vi "Point+Scan .vi"() -> ()   [LabVIEW 2014]
doc: "This is the main user interface of the Raman spectroscopy system."
uses:
  <userlib>/atmcd64d.llb/AcquisitionMode_mode typedef.ctl
  <userlib>/atmcd64d.llb/ReadMode_mode typedef.ctl
  <userlib>/atmcd64d.llb/Shutter_mode typedef.ctl
  <userlib>/atmcd64d.llb/Shutter_type typedef.ctl
  <userlib>/atmcd64d.llb/TriggerMode_mode typedef.ctl
  TypeDef/GalvoInput.ctl
  <userlib>/atmcd64d.llb/Error Code Enum typedef.ctl
  TypeDef/States.ctl
panel:
  in  "Tab Control":enum32{"Main", "Andor", "Galvo"}(tab)
  in  "Scan Range":T1={"Ver_V/H"=0.070604, "Hor_V/W"=0.086202, "Ver_r/p"=4.0, "Hor_r/p"=4.0}
  in  "Scan Resolusion":T2={"Ver_V"=0.17651, "Hor_H"=0.2155, "Ver_Pix"=471.9764, "Hor_Pix"=471.9764}
  in  "Galvo Center":bool
  out "Galvo":bool
  in  "Quit":bool
  out "Initialization finished":bool
  in  "Galvo Stop":bool
  in  "Galvo Scan":bool
  out "Andor":bool
  out "CurrentFrame":i32
  out "H":i32
  out "V":i32
  in  "Set":bool
  in  "AndorSnap":bool
  out "SaveStatus":bool
  in  "FilePath":string="C:\\Users\\light\\Desktop\\SI+Raman\\data\\TEMP"
  in  "Exit":bool
  out "ShutDown":cluster{"CoolOff":bool, "ShutDown":bool}
  in  "Mode":T8={"AcqMode"=enum."Single Scan", "ReadMode"=enum."Single-Track", "ShutterMode"=enum."Auto", "GateMode"=enum."TTL High", "TriggerMode"=enum."Internal"}
  in  "AcqSet":T9={"openingtime"=0, "closingtime/ms"=0, "ExposureTime/s"=0.1, "AccumCycTime"=0.0, "AccumCycNum"=1, "KineticNum"=1, "KineticTime"=0.0} {"KineticTime" format="%.5f"; "AccumCycNum" format="%.5f"; "AccumCycTime" format="%.5f"; "ExposureTime/s" format="%.5f"; "closingtime/ms" format="%.2f"; "openingtime" format="%.2f"}
  out "Timing":T10 {"kinetic" format="%.7f"; "accumulate" format="%.7f"; "exposure" format="%.7f"}
  out "SetOut":T11
  in  "MultiTrack":cluster{"StartRow":i32, "EndRow":i32}={"StartRow"=122, "EndRow"=133}
  out "SetStatus":bool
  out "CurrentTemp":i32
  out "DevInit":bool
  out "DevSize":cluster{"xpixels":i32, "ypixels":i32}
  out "HardWVersion":T12
  out "SoftWVersion":T13
  out "Speeds":T14
  in  "TargetTemp":i32=-60
  out "CoolerON":T15
  out "GetStatus":T16
  in  "YOffset":dbl=5.75 caption="Offset"
  in  "XOffset":dbl=3.1 caption="Offset"
  out "Sample Rate":dbl=1000.0 format="%0.2f"
  out "Waveform Graph":waveform(dbl)[](graph)=[{"t0"=timestamp(0 s since 1904-01-01), "dt"=0.001, "Y"=[]}]
  in  "ZOffset":dbl=1.6 caption="Offset"
  in  "Galvo":T17={"Sample Rate"=100000.0, "Sample Clock Source"="OnboardClock", "Max Voltage"=10.0, "Min Voltage"=-10.0, "Physical Channel(s)"="Dev1/ao0,Dev1/ao1,Dev1/ao3"}
  # "Objective: CFI Plan Fluor ELWD 60x (1.27 NA) \nThe depth of field: 1.78 um\nPixel Size: 0.0877um/px"
  # "Kinetics->SignleTrack"
  # "Galvo Control"
  # "50Hz->1s"
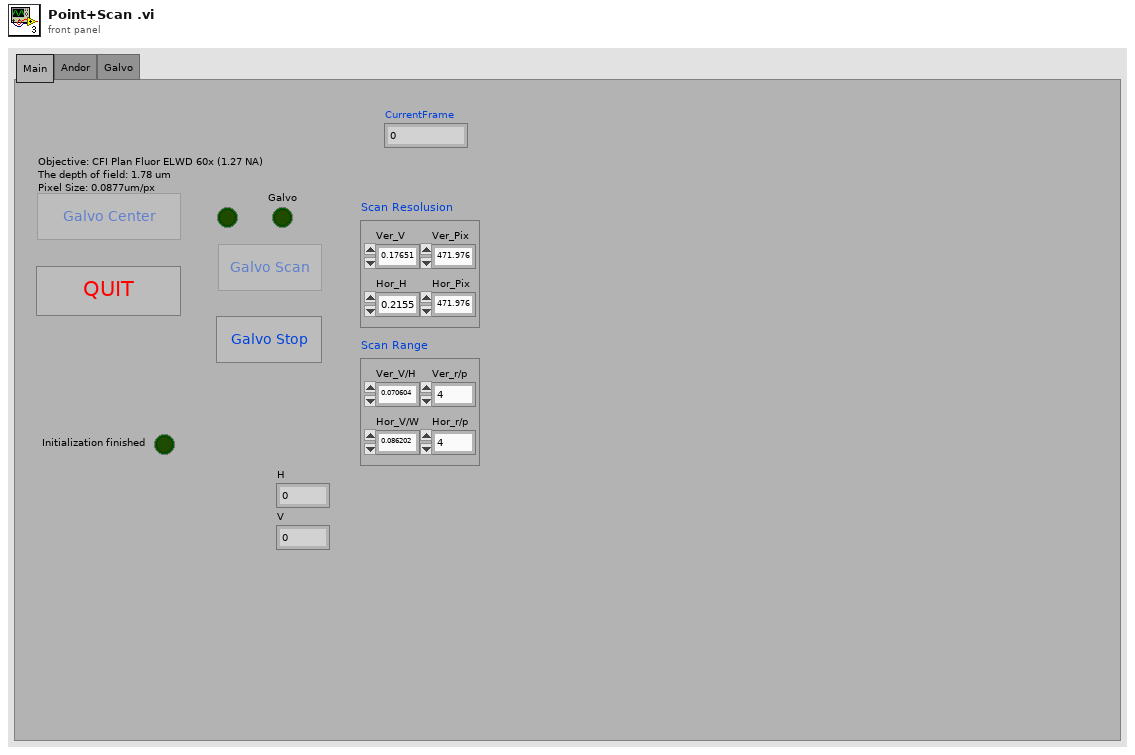
[diagram p1: front panel]
types:
  T1 = cluster{"Ver_V/H":dbl, "Hor_V/W":dbl, "Ver_r/p":dbl, "Hor_r/p":dbl}
  T2 = cluster{"Ver_V":dbl, "Hor_H":dbl, "Ver_Pix":dbl, "Hor_Pix":dbl}
  T3 = typedef "AcquisitionMode_mode typedef.ctl" = enum16{"Reserved (0)", "Single Scan", "Accumulate", "Kinetics", "Fast Kinetics", "Run Till Abort", "Reserved (6)", "Reserved (7)", "Reserved (8)", "Time Delayed Integration"}
  T4 = typedef "ReadMode_mode typedef.ctl" = enum16{"Full Vertical Binning", "Multi-Track", "Random-Track", "Single-Track", "Image"}
  T5 = typedef "Shutter_mode typedef.ctl" = enum16{"Auto", "Open", "Close", "N/A (3)", "Open FVB Series", "Open Any Series"}
  T6 = typedef "Shutter_type typedef.ctl" = enum16{"TTL Low", "TTL High"}
  T7 = typedef "TriggerMode_mode typedef.ctl" = enum16{"Internal", "External", "N/A (2)", "N/A (3)", "N/A (4)", "N/A (5)", "External Start", "External Exposure (Bulb)", "N/A (8)", "External FVB EM", "Software", "N/A (11)", "External Charge Shifting"}
  T8 = cluster{"AcqMode":T3, "ReadMode":T4, "ShutterMode":T5, "GateMode":T6, "TriggerMode":T7}
  T9 = cluster{"openingtime":i32, "closingtime/ms":i32, "ExposureTime/s":sgl, "AccumCycTime":sgl, "AccumCycNum":i32, "KineticNum":i32, "KineticTime":sgl}
  T10 = cluster{"exposure":sgl, "accumulate":sgl, "kinetic":sgl}
  T11 = cluster{"Height":i32, "Width":i32, "bottom":i32, "gap":i32}
  T12 = cluster{"PCB":u32, "Flex":u32, "dummy1":u32, "dummy2":u32, "dummy3":u32, "dummy4":u32}
  T13 = cluster{"eprom":u32, "cofFile":u32, "vxdRev":u32, "vxdVer":u32, "dllRev":u32, "dllVer":u32}
  T14 = cluster{"NVS":i32, "VS":i32, "NHS":dbl, "HS":i32}
  T15 = cluster{"SetTemp":bool, "CoolerOn":bool, "Stablized":bool}
  T16 = cluster{"GetDetector":bool, "GetHardVer":bool, "GetNVS":bool, "GetVS":bool, "GetSotfVer":bool, "GetNHS":bool, "GetHS":bool}
  T17 = typedef "GalvoInput.ctl" = cluster{"Sample Rate":dbl, "Sample Clock Source":tag, "Max Voltage":dbl, "Min Voltage":dbl, "Physical Channel(s)":tag}
  T18 = typedef "States.ctl" = enum16{"Initialize", "CMOS live", "Shut down"}
  T19 = enum8{"Enabled", "Disabled", "Disabled and Grayed Out"}
  T20 = typedef "Error Code Enum typedef.ctl" = enum32{"N/A (0)", "DRV_ERROR_CODES", "DRV_SUCCESS", "DRV_VXDNOTINSTALLED", "DRV_ERROR_SCAN", "DRV_ERROR_CHECK_SUM", "DRV_ERROR_FILELOAD", "DRV_UNKNOWN_FUNC", "DRV_ERROR_VXD_INIT", "DRV_ERROR_ADDRESS", "DRV_ERROR_PAGELOCK", "DRV_ERROR_PAGEUNLOCK", "DRV_ERROR_BOARDTEST", "DRV_ERROR_ACK", "DRV_ERROR_UP_FIFO", "DRV_ERROR_PATTERN", "N/A (16)", "DRV_ACQUISITION_ERRORS", "DRV_ACQ_BUFFER", "DRV_ACQ_DOWNFIFO_FULL", "DRV_PROC_UNKONWN_INSTRUCTION", "DRV_ILLEGAL_OP_CODE", "DRV_KINETIC_TIME_NOT_MET", "DRV_ACCUM_TIME_NOT_MET", "DRV_NO_NEW_DATA", "N/A (25)", "DRV_SPOOLERROR", "N/A (27)", "N/A (28)", "N/A (29)", "N/A (30)", "N/A (31)", "N/A (32)", "DRV_TEMPERATURE_CODES", "DRV_TEMPERATURE_OFF", "DRV_TEMPERATURE_NOT_STABILIZED", "DRV_TEMPERATURE_STABILIZED", "DRV_TEMPERATURE_NOT_REACHED", "DRV_TEMPERATURE_OUT_RANGE", "DRV_TEMPERATURE_NOT_SUPPORTED", "DRV_TEMPERATURE_DRIFT", "N/A (41)", "N/A (42)", "N/A (43)", "N/A (44)", "N/A (45)", "N/A (46)", "N/A (47)", "N/A (48)", "DRV_GENERAL_ERRORS", "DRV_INVALID_AUX", "DRV_COF_NOTLOADED", "DRV_FPGAPROG", "DRV_FLEXERROR", "DRV_GPIBERROR", "N/A (55)", "N/A (56)", "N/A (57)", "N/A (58)", "N/A (59)", "N/A (60)", "N/A (61)", "N/A (62)", "N/A (63)", "DRV_DATATYPE", "DRV_DRIVER_ERRORS", "DRV_P1INVALID", "DRV_P2INVALID", "DRV_P3INVALID", "DRV_P4INVALID", "DRV_INIERROR", "DRV_COFERROR", "DRV_ACQUIRING", "DRV_IDLE", "DRV_TEMPCYCLE", "DRV_NOT_INITIALIZED", "DRV_P5INVALID", "DRV_P6INVALID", "DRV_INVALID_MODE", "DRV_INVALID_FILTER", "DRV_I2CERRORS", "DRV_I2CDEVNOTFOUND", "DRV_I2CTIMEOUT", "DRV_P7INVALID", "N/A (84)", "N/A (85)", "N/A (86)", "N/A (87)", "N/A (88)", "N/A (89)", "DRV_IOCERROR", "DRV_VRMVERSIONERROR"}
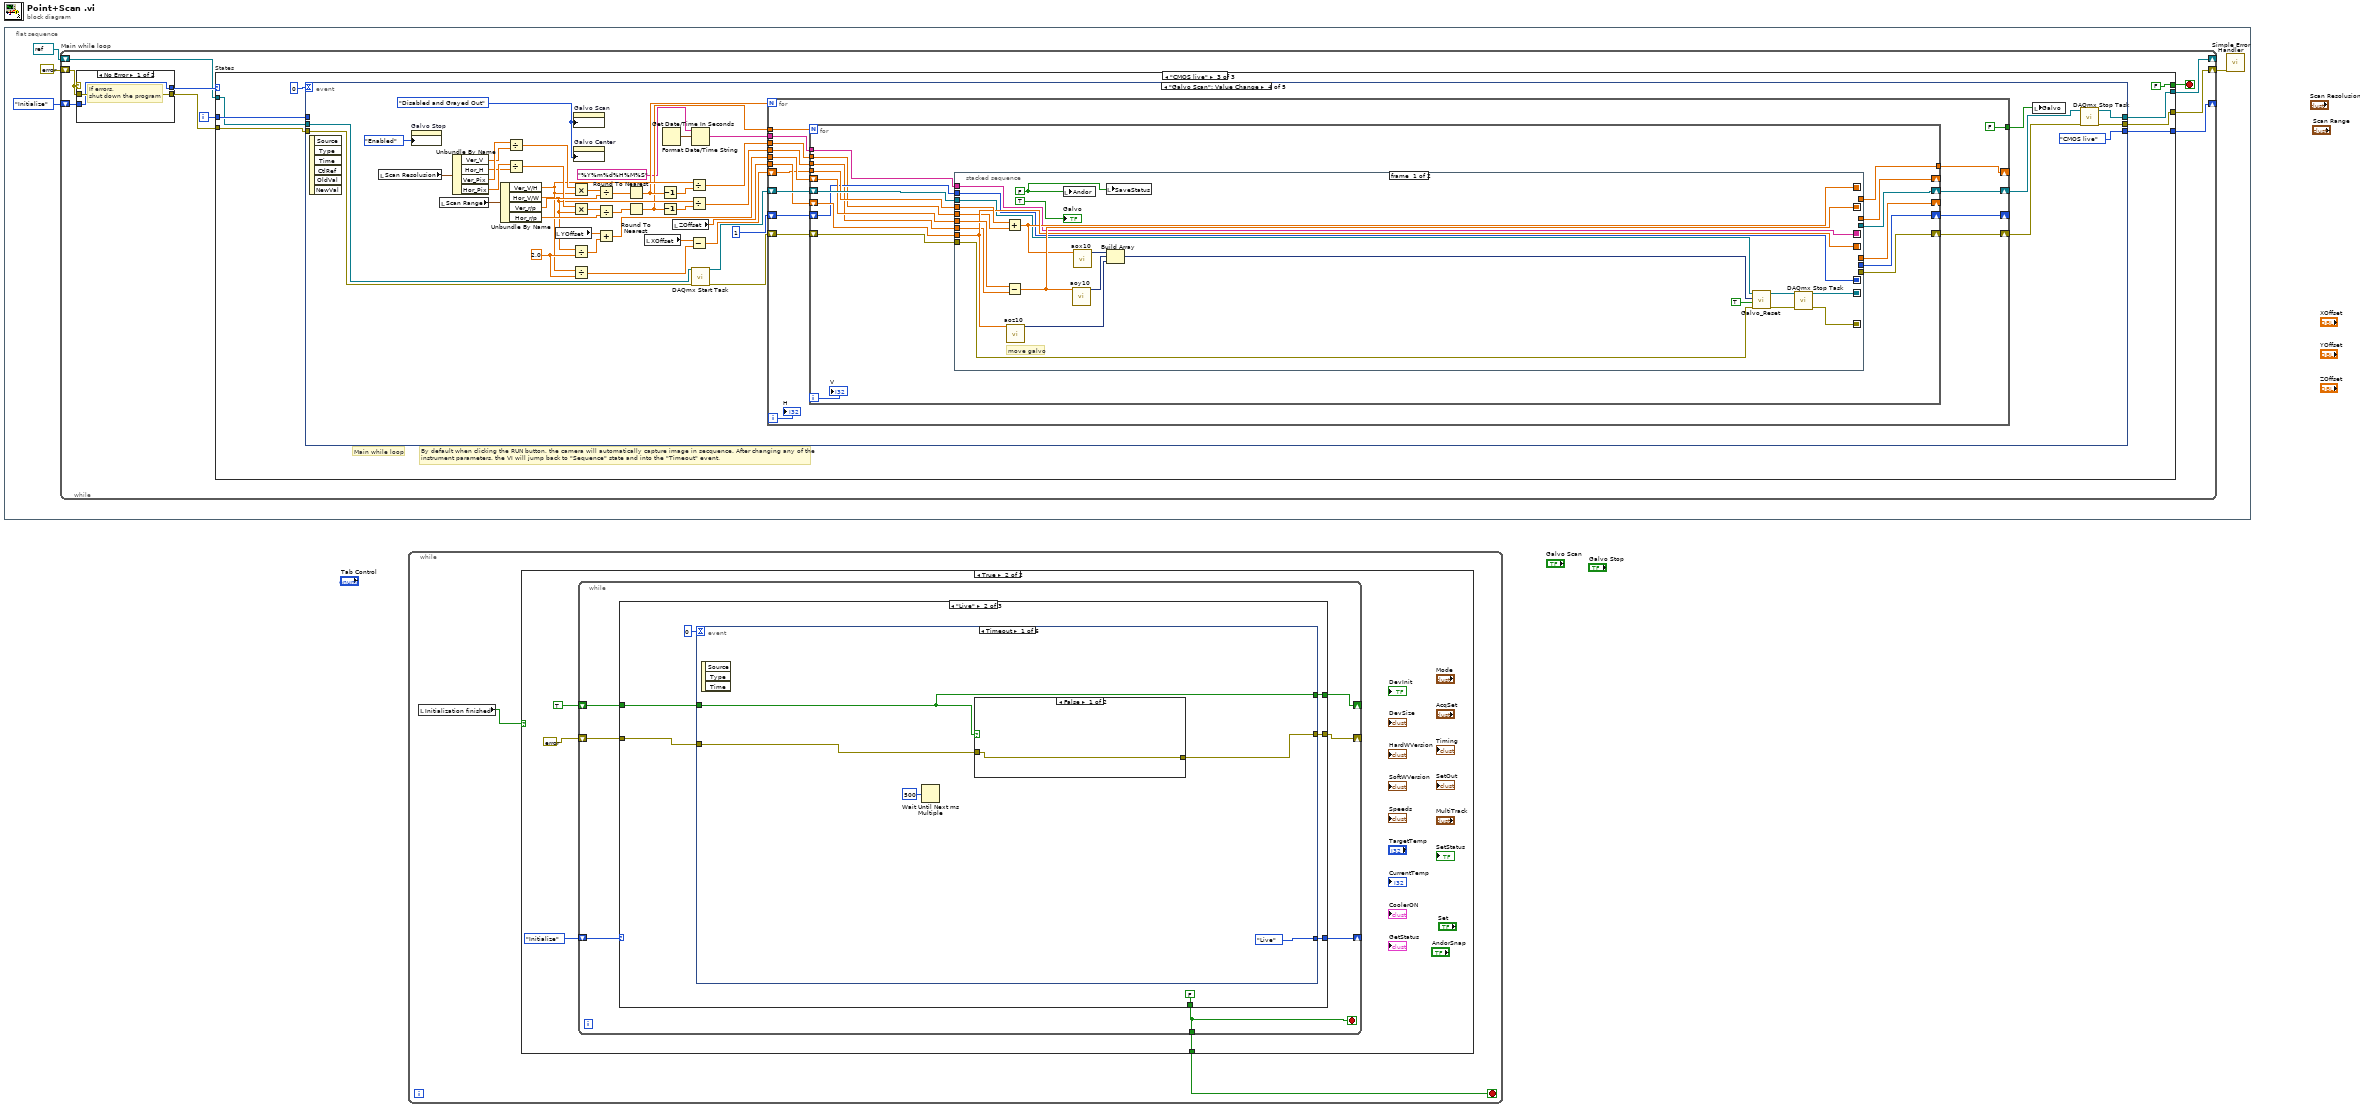
[diagram p0: block diagram]
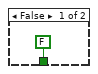
[diagram p2: hidden frame]
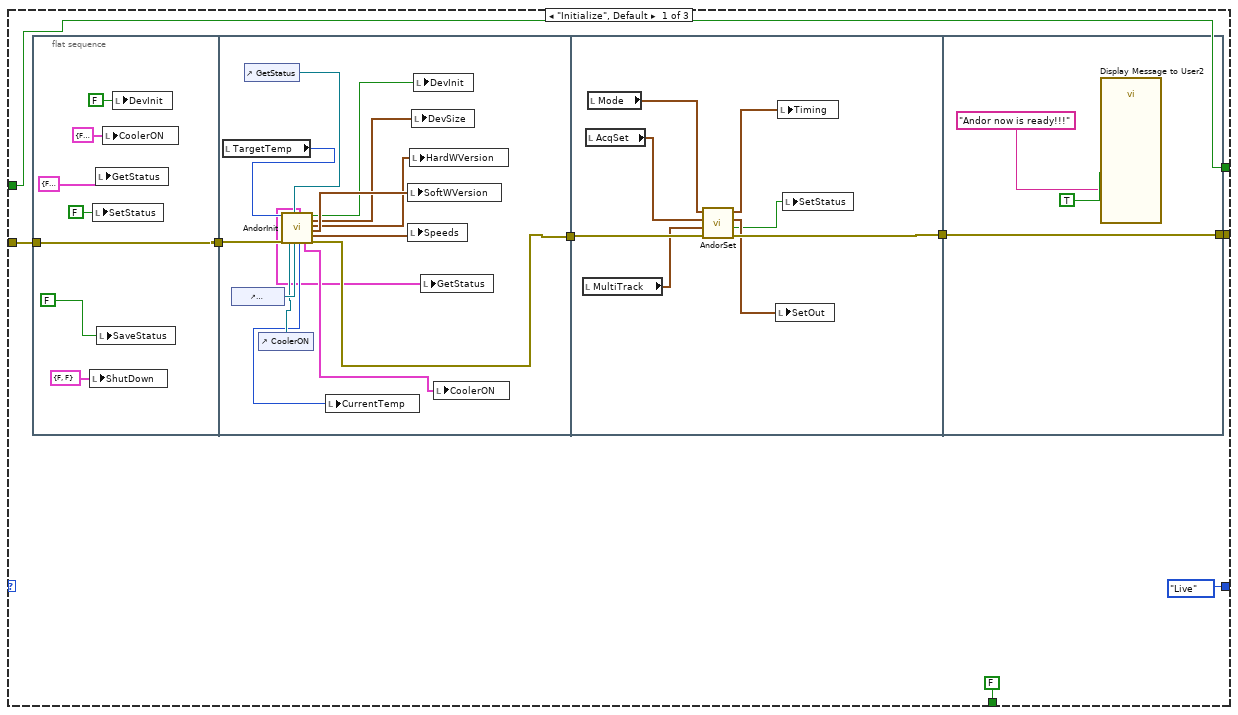
[diagram p3: hidden frame]
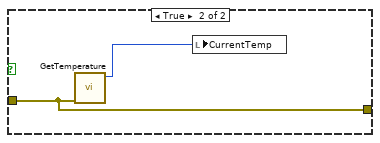
[diagram p4: hidden frame]
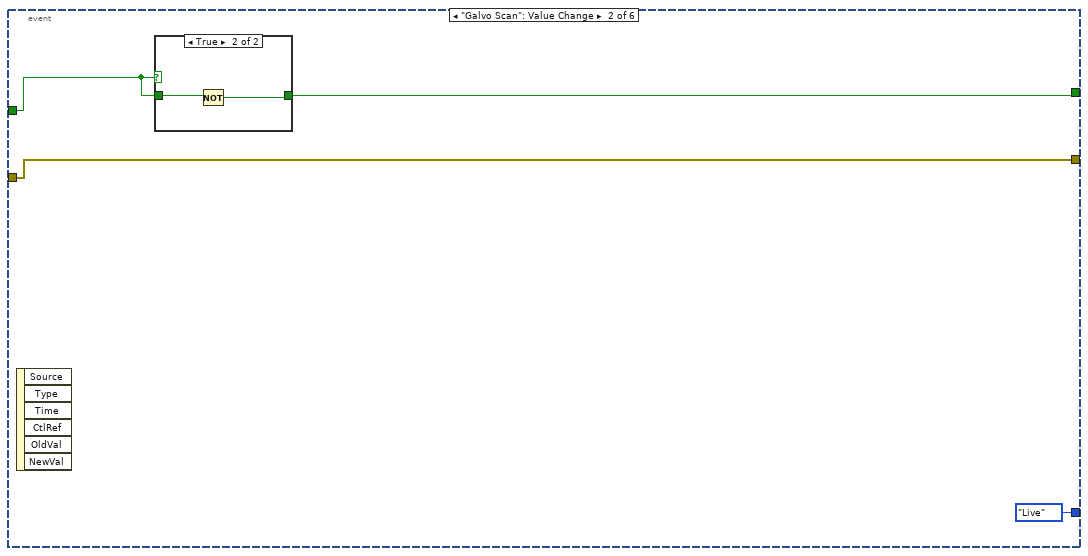
[diagram p5: hidden frame]
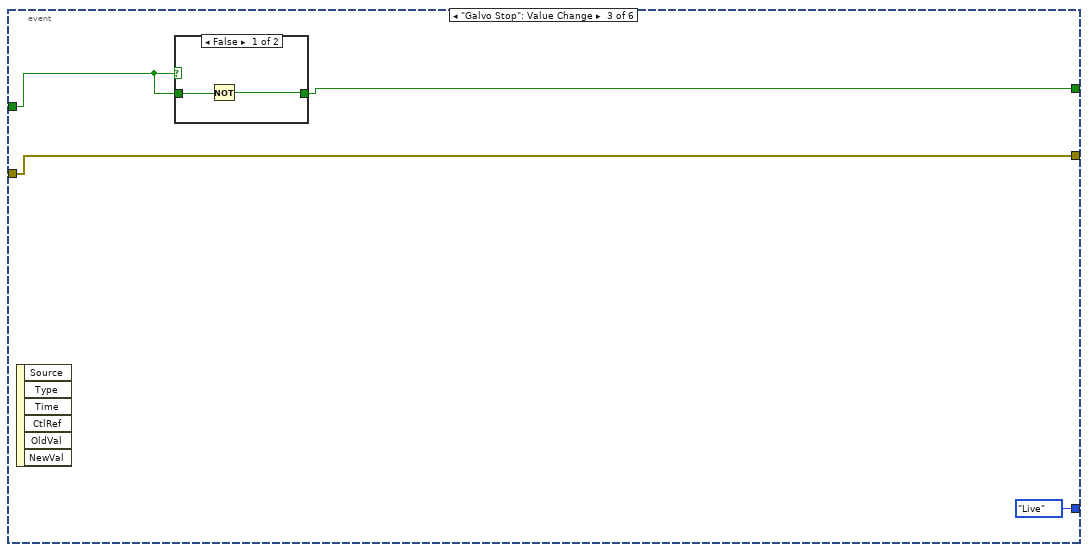
[diagram p7: hidden frame]
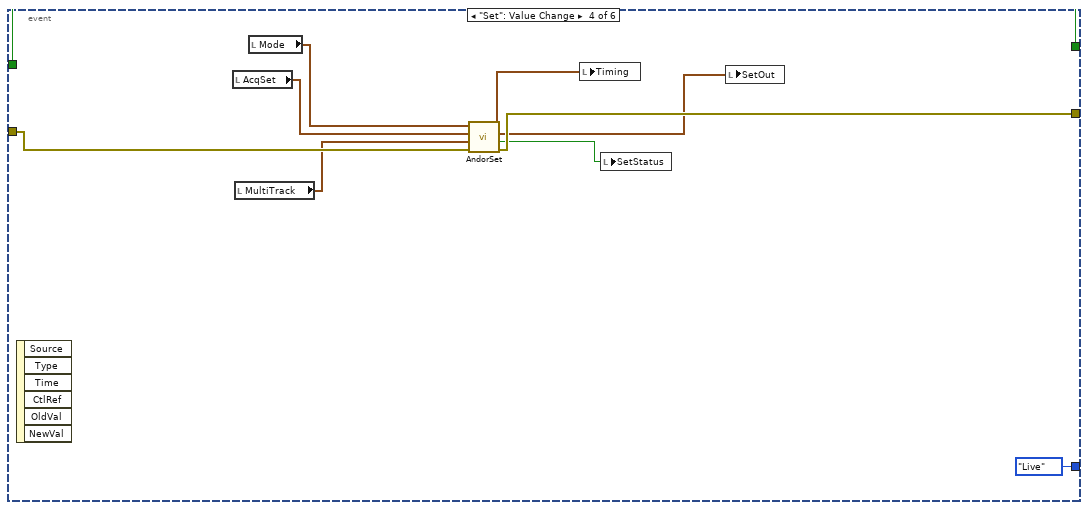
[diagram p9: hidden frame]
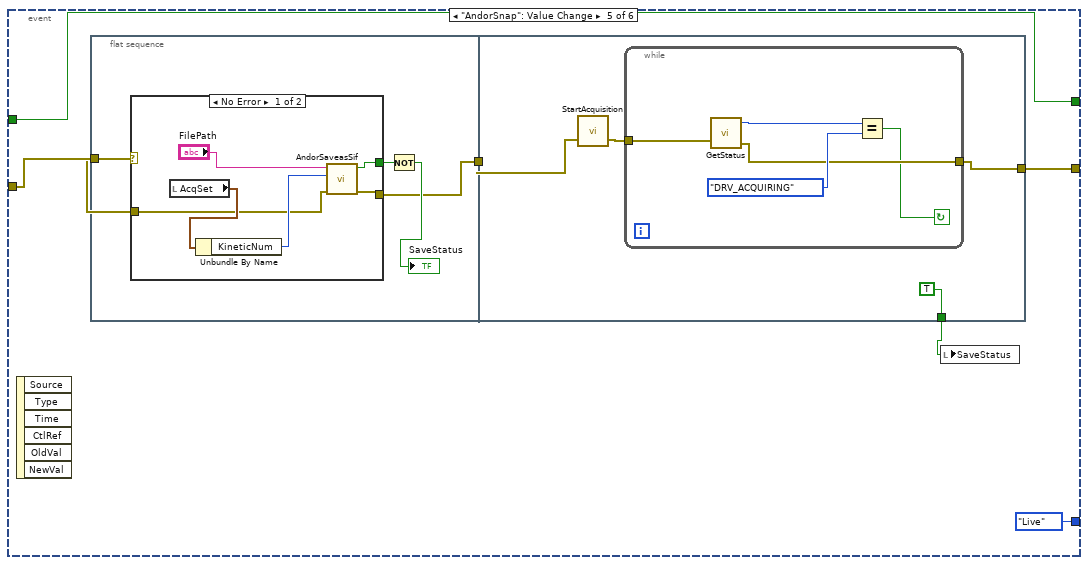
[diagram p10: hidden frame]
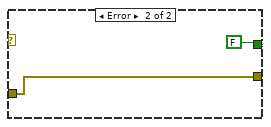
[diagram p11: hidden frame]
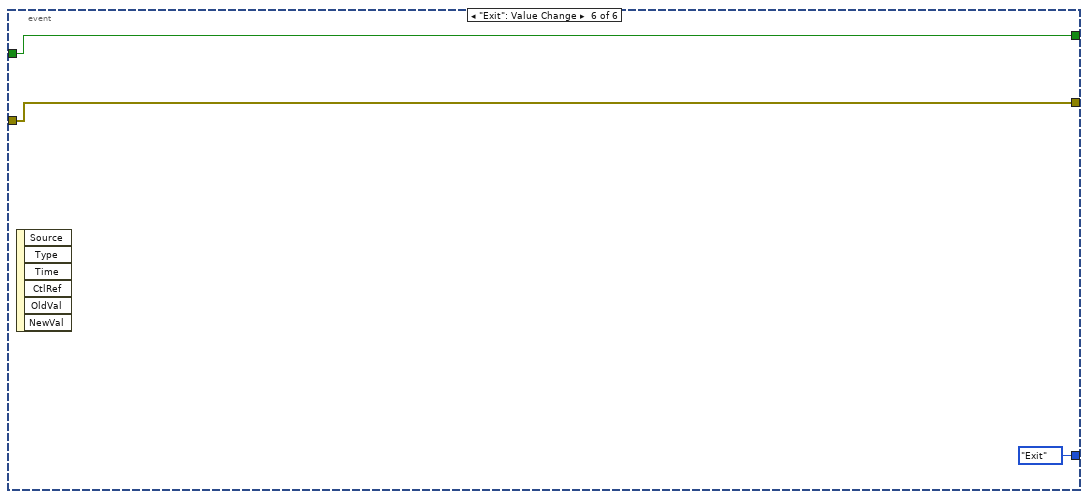
[diagram p12: hidden frame]
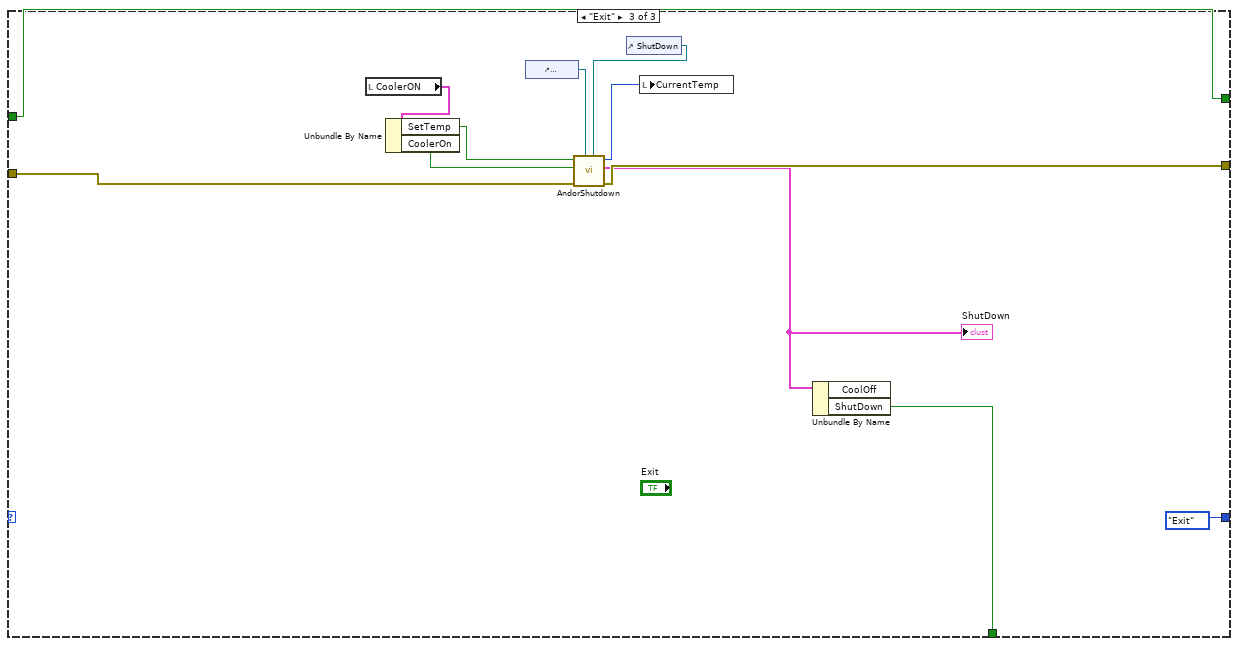
[diagram p13: hidden frame]
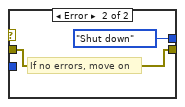
[diagram p14: hidden frame]
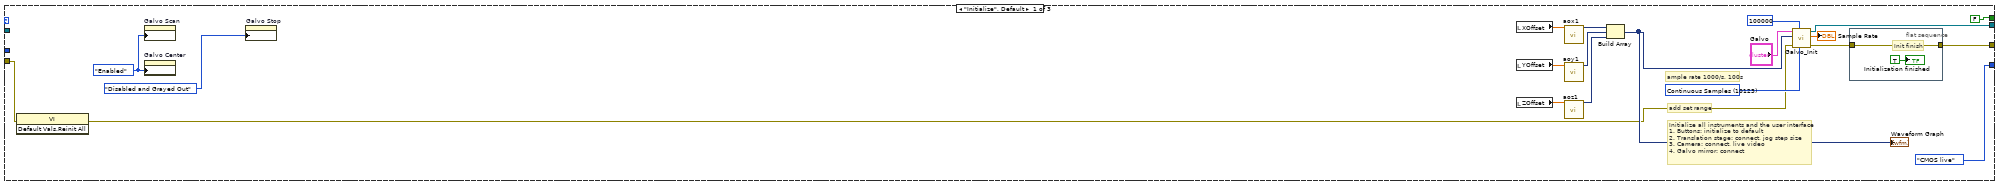
[diagram p15: hidden frame]
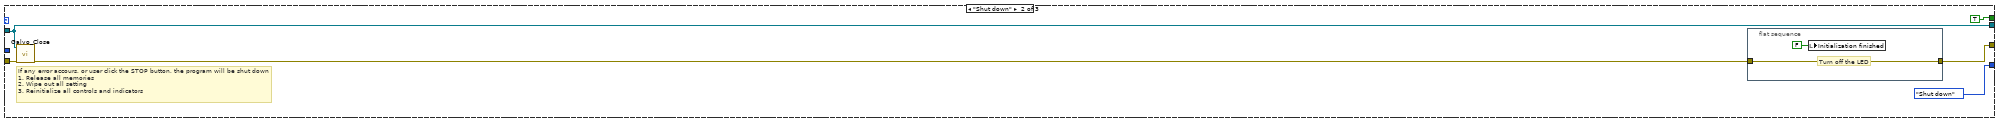
[diagram p16: hidden frame]
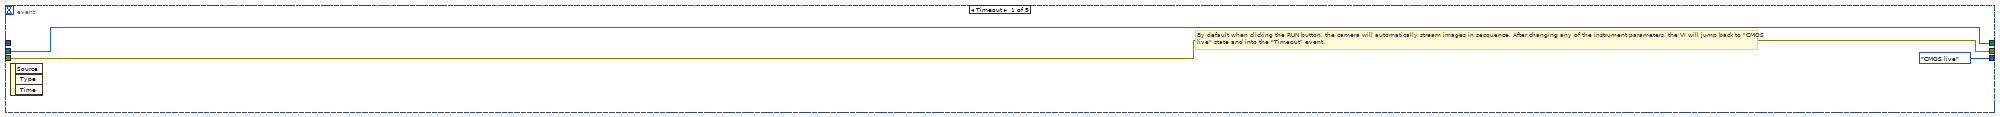
[diagram p17: hidden frame]
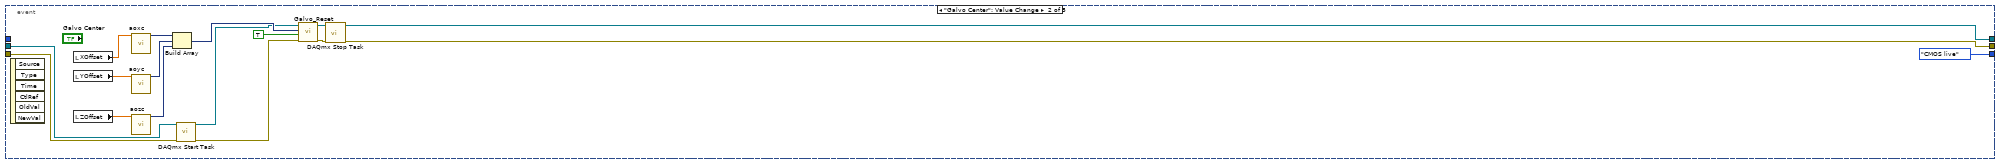
[diagram p18: hidden frame]
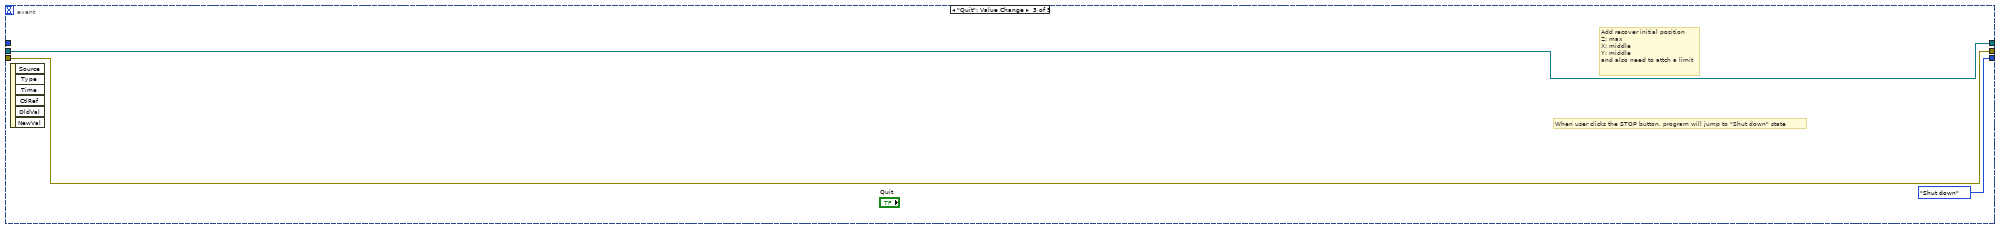
[diagram p19: hidden frame]
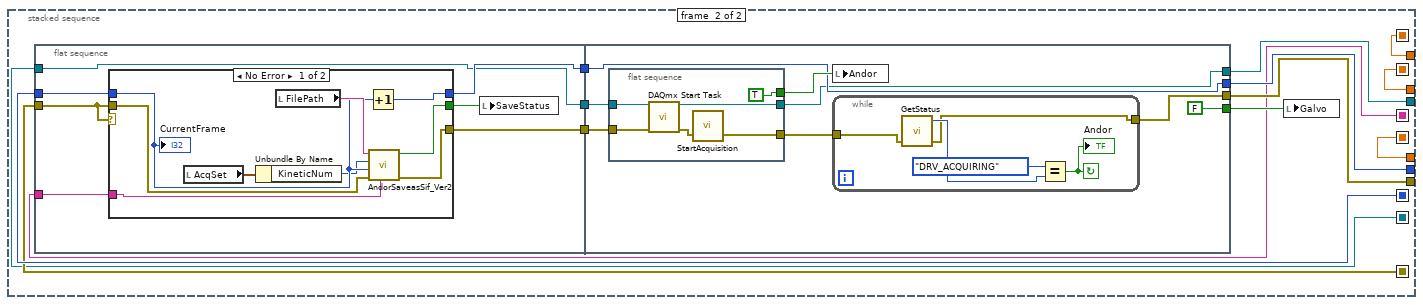
[diagram p20: hidden frame]
diagram:
  n1 = flat-sequence {
    frame #0 {
      n2 = while "Main while loop" {
        shift-right: [w9] -> _
        shift-left: States."Initialize" -> [w14]
        shift-right: [w12] -> w2
        shift-left: errorcluster {"status"=FALSE, "code"=0, "source"=""} ("error out") -> [w8]
        shift-right: [w6] -> _
        shift-left: refnum<k21> refnum ("task out") -> [w5]
        i -> [w7]
        stop <- w10 stop-if-true
        n3 = case shown="No Error" w8 {
          tunnel: w8 -> [w16 w18]
          tunnel: [w16 w18] -> w11
          tunnel: w14 -> [w15 _]
          tunnel: [w15 States."Shut down"] -> w13
          frame No Error {
            # "If errors,\nshut down the program"
          }
          frame Error {
            # "If no errors, move on"
          }
        }
        n4 = case "States" shown="\"CMOS live\"" w13 {
          tunnel: [w36 w41 w54] -> w12
          tunnel: w11 -> [w37 w42 w55]
          tunnel: [FALSE TRUE FALSE] -> w10
          tunnel: [States."CMOS live" States."Shut down" w56] -> w9
          tunnel: w7 -> [_ _ w52]
          tunnel: [w33 w44 w50] -> w6
          tunnel: w5 -> [_ w44 w51]
          frame "Initialize", Default {
            w22 = T19."Enabled" ("Disabled")
            w28 = 10123 items=["Finite Samples"=10178, "Continuous Samples"=10123, "Hardware Timed Single Point"=12522] ("Sample Mode")
            # "ample rate 1000/s, 100s"
            # "add set range"
            # "Initialize all instruments and the user interface\n1. Buttons: initialize to default\n2. Translation stage: connect, jog step size\n3. Camera: connect, live video\n4. Galvo mirror: connect"
            n5 = invoke class="VI" method="Default Vals.Reinit All"(error in=w37) -> (error out=w21:errorcluster)  [unwired: 2 in, 2 out]
            n6 = property on="Galvo Scan" class="Bool"("DisabledEnum"=w22) -> ()  [unwired: 2 in, 2 out]
            n7 = property on="Galvo Center" class="Bool"("DisabledEnum"=w22) -> ()  [unwired: 2 in, 2 out]
            n8 = property on="Galvo Stop" class="Bool"("DisabledEnum"=T19."Disabled and Grayed Out" ("Disabled")) -> ()  [unwired: 2 in, 2 out]
            n9 = local read "XOffset"() -> (w25:dbl)
            n10 = local read "YOffset"() -> (w24:dbl)
            n11 = local read "ZOffset"() -> (w23:dbl)
            n12 = call "aox1"("Offset"=w25) -> ("DC"=w27:dynamicdata)  [unwired: 13 in, 1 out]
            n13 = call "aoy1"("Offset"=w24) -> ("DC"=w26:dynamicdata)  [unwired: 13 in, 1 out]
            n14 = call "aoz1"("Offset"=w23) -> ("DC"=w31:dynamicdata)  [unwired: 13 in, 1 out]
            n15 = Build Array(w27, w26, w31) -> (w30:dynamicdata[])
            "Waveform Graph" <- w30
            n16 = call "Galvo_Init.vi"("Sample Mode"=w28, "samples per channel"=100000, "error in"=w21, "Signal array"=w30, "Galvo_Input"="Galvo") -> ("error out"=w32:errorcluster, "Actual Sample Rate"=→"Sample Rate":dbl, "task out"=w33:refnum<k21>)  [unwired: 4 in]
            n17 = flat-sequence {
              tunnel: w32 -> [w40]
              tunnel: [w40] -> w36
              frame #0 {
                # "Init finish"
                "Initialization finished" <- TRUE ("Initialization finished")
              }
            }
          }
          frame "Shut down" {
            # "If any error accours, or user click the STOP button, the program will be shut down\n1. Release all memories\n2. Wipe out all setting\n3. Reinitialize all controls and indicators"
            n18 = call "Galvo_Close.vi"("error in"=w42, "task/channels in"=w44) -> ("error out"=w43:errorcluster)  [unwired: 9 in]
            n19 = flat-sequence {
              tunnel: w43 -> [w47]
              tunnel: [w47] -> w41
              frame #0 {
                # "Turn off the LED"
                n20 = local write "Initialization finished"(FALSE ("Initialization finished")) -> ()
              }
            }
          }
          frame "CMOS live" {
            # "Main while loop"
            # "By default when clicking the RUN button, the camera will automatically capture image in secquence. After changing any of the \ninstrument parameters, the VI will jump back to \"Sequence\" state and into the \"Timeout\" event."
            n21 = event shown="[3] \"Galvo Scan\": Value Change" {
              selector: _ -> [_ _ _ _ _]
              dyn-events: _ -> [_ _ _ _ _]
              timeout: 0 -> [_ _ _ _ _]
              tunnel: [States."CMOS live" States."CMOS live" States."Shut down" States."CMOS live" States."CMOS live"] -> w56
              tunnel: w55 -> [w57 w68 w78 w82 w232]
              tunnel: [w57 w62 w78 w109 w232] -> w54
              tunnel: w52 -> [_ _ _ _ _]
              tunnel: [w59 w63 w77 w108 w234] -> w50
              tunnel: w51 -> [w59 w70 w77 w124 w234]
              event Timeout {
                # "By default when clicking the RUN button, the camera will automatically stream images in secquence. After changing any of the instrument parameters, the VI will jump back to \"CMOS live\" state and into the \"Timeout\" event."
                n22 = event-data() -> ()  [unwired: 1 in, 3 out]
              }
              event "Galvo Center": Value Change {
                n23 = event-data() -> ()  [unwired: 1 in, 6 out]
                n24 = local read "XOffset"() -> (w61:dbl)
                n25 = local read "YOffset"() -> (w60:dbl)
                n26 = local read "ZOffset"() -> (w74:dbl)
                n27 = call "aoxc"("Offset"=w61) -> ("DC"=w72:dynamicdata)  [unwired: 13 in, 1 out]
                n28 = call "aoyc"("Offset"=w60) -> ("DC"=w71:dynamicdata)  [unwired: 13 in, 1 out]
                n29 = call "aozc"("Offset"=w74) -> ("DC"=w75:dynamicdata)  [unwired: 13 in, 1 out]
                n30 = Build Array(w72, w71, w75) -> (w73:dynamicdata[])
                n31 = call <vilib>:"DAQmx Start Task.vi"("task/channels in"=w70, "error in"=w68) -> ("task out"=w69:refnum<k21>, "error out"=w67:errorcluster)  [unwired: 12 in]
                n32 = call "Galvo_Reset.vi"("error in"=w67, "auto start"=TRUE, "Signal array"=w73, "task/channels in"=w69) -> ("error out"=w64:errorcluster, "task out"=w65:refnum<k21>)  [unwired: 6 in]
                n33 = call <vilib>:"DAQmx Stop Task.vi"("task/channels in"=w65, "error in"=w64) -> ("task out"=w63:refnum<k21>, "error out"=w62:errorcluster)  [unwired: 12 in]
              }
              event "Quit": Value Change {
                # "Add recover initial position\nZ: max\nX: middle\nY: middle\nand also need to attch a limit"
                # "When user clicks the STOP button, program will jump to \"Shut down\" state"
                n34 = event-data() -> ()  [unwired: 1 in, 6 out]
              }
              event "Galvo Scan": Value Change {
                w107 = 2.0 ("y")
                w80 = T19."Disabled and Grayed Out" ("Disabled")
                n35 = event-data() -> ()  [unwired: 1 in, 6 out]
                n36 = local read "Scan Resolusion"() -> (w123:T2)
                n37 = property on="Galvo Stop" class="Bool"("DisabledEnum"=T19."Enabled" ("Disabled")) -> ()  [unwired: 2 in, 2 out]
                n38 = local read "Scan Range"() -> (w120:T1)
                n39 = Unbundle By Name(w123) -> ("Ver_V"=w121:dbl, "Hor_H"=w94:dbl, "Ver_Pix"=w122:dbl, "Hor_Pix"=w95:dbl)
                n40 = Unbundle By Name(w120) -> ("Ver_V/H"=w93:dbl, "Hor_V/W"=w92:dbl, "Ver_r/p"=w118:dbl, "Hor_r/p"=w116:dbl)
                n41 = Divide(x=w122, y=w121) -> (x/y=w99:dbl)
                n42 = Divide(x=w95, y=w94) -> (x/y=w98:dbl)
                n43 = local read "YOffset"() -> (w104:dbl)
                n44 = Multiply(x=w99, y=w93) -> (x*y=w119:dbl)
                n45 = Multiply(x=w98, y=w92) -> (x*y=w117:dbl)
                n46 = Divide(x=w92, y=w107) -> (x/y=w103:dbl)
                n47 = Divide(x=w93, y=w107) -> (x/y=w105:dbl)
                n48 = property on="Galvo Scan" class="Bool"("DisabledEnum"=w80) -> ()  [unwired: 2 in, 2 out]
                n49 = property on="Galvo Center" class="Bool"("DisabledEnum"=w80) -> ()  [unwired: 2 in, 2 out]
                n50 = Divide(x=w119, y=w118) -> (x/y=w115:dbl)
                n51 = Divide(x=w117, y=w116) -> (x/y=w96:dbl)
                n52 = Add(x=w104, y=w103) -> (x+y=w101:dbl)
                n53 = Round To Nearest(number=w115) -> (nearest integer value=w91:dbl)
                n54 = Round To Nearest(number=w96) -> (nearest integer value=w89:dbl)
                n55 = local read "XOffset"() -> (w106:dbl)
                n56 = Decrement(x=w91) -> (x-1=w90:dbl)
                n57 = Decrement(x=w89) -> (x-1=w88:dbl)
                n58 = Get Date/Time In Seconds() -> (seconds since 1Jan1904=w85:timestamp)
                n59 = local read "ZOffset"() -> (w100:dbl)
                n60 = Divide(x=w93, y=w90) -> (x/y=w87:dbl)
                n61 = Divide(x=w92, y=w88) -> (x/y=w86:dbl)
                n62 = Subtract(x=w106, y=w105) -> (x-y=w102:dbl)
                n63 = Format Date/Time String(time format string (%c)="%Y%m%d%H%M%S", seconds (now)=w85) -> (date/time string=w83:string)  [unwired: 1 in]
                n64 = call <vilib>:"DAQmx Start Task.vi"("task/channels in"=w124, "error in"=w82) -> ("task out"=w112:refnum<k21>, "error out"=w114:errorcluster)  [unwired: 12 in]
                n65 = for {
                  N: w91 -> [_]
                  tunnel: [FALSE ("Galvo")] -> w113
                  shift-right: [w140] -> w110
                  shift-left: w114 -> [w139]
                  shift-right: [w133] -> _
                  shift-left: w102 -> [w134]
                  shift-right: [w137] -> w111
                  shift-left: w112 -> [w138]
                  tunnel: w101 -> [w136]
                  tunnel: w100 -> [w135]
                  shift-right: [w131] -> _
                  shift-left: 1 -> [w132]
                  tunnel: w89 -> [w130]
                  tunnel: w87 -> [w129]
                  tunnel: w86 -> [w128]
                  tunnel: w83 -> [w127]
                  i -> [w126]
                  n66 = for {
                    N: w130 -> [_]
                    shift-right: [w147] -> w140
                    shift-left: w139 -> [w157]
                    shift-right: [w145] -> _
                    shift-left: w136 -> [w154]
                    shift-right: [w146] -> _
                    shift-left: w135 -> [w153]
                    shift-right: [w148] -> w137
                    shift-left: w138 -> [w156]
                    tunnel: w134 -> [w155]
                    tunnel: [w144] -> w133
                    shift-right: [w143] -> w131
                    shift-left: w132 -> [w152]
                    tunnel: w129 -> [w151]
                    tunnel: w128 -> [w150]
                    tunnel: w127 -> [w149]
                    i -> [w142]
                    n67 = stacked-sequence {
                      seq-local: [w164 _] -> [_ w184]
                      seq-local: [w170 _] -> [_ w187]
                      seq-local: [w169 _] -> [_ w186]
                      seq-local: [w168 _] -> [_ w185]
                      seq-local: [w162 _] -> [_ w192]
                      seq-local: [w161 _] -> [_ w183]
                      seq-local: [w158 _] -> [_ w182]
                      tunnel: w157 -> [w171 _]
                      tunnel: w156 -> [w160 _]
                      tunnel: w155 -> [w173 _]
                      tunnel: w154 -> [w172 _]
                      tunnel: w153 -> [w169 _]
                      tunnel: w152 -> [w162 _]
                      tunnel: w151 -> [w167 _]
                      tunnel: w150 -> [w166 _]
                      tunnel: w149 -> [w161 _]
                      tunnel: [_ w187] -> w145
                      tunnel: [_ w186] -> w146
                      tunnel: [_ w185] -> w144
                      tunnel: [_ w190] -> w143
                      tunnel: [_ w189] -> w147
                      tunnel: [_ w180] -> w148
                      frame #0 {
                        w176 = FALSE ("SaveStatus")
                        # "move galvo"
                        n68 = Add(x=w173, y=w167) -> (x+y=w168:dbl)
                        n69 = Subtract(x=w172, y=w166) -> (x-y=w170:dbl)
                        n70 = call "aoz10"("Offset"=w169) -> ("DC"=w179:dynamicdata)  [unwired: 13 in, 1 out]
                        n71 = local write "Andor"(w176) -> ()
                        n72 = call "aoy10"("Offset"=w170) -> ("DC"=w177:dynamicdata)  [unwired: 13 in, 1 out]
                        n73 = call "aox10"("Offset"=w168) -> ("DC"=w178:dynamicdata)  [unwired: 13 in, 1 out]
                        n74 = local write "SaveStatus"(w176) -> ()
                        n75 = Build Array(w178, w177, w179) -> (w174:dynamicdata[])
                        n76 = call "Galvo_Reset.vi"("error in"=w171, "auto start"=TRUE, "Signal array"=w174, "task/channels in"=w160) -> ("error out"=w165:errorcluster, "task out"=w159:refnum<k21>)  [unwired: 6 in]
                        n77 = call <vilib>:"DAQmx Stop Task.vi"("task/channels in"=w159, "error in"=w165) -> ("task out"=w158:refnum<k21>, "error out"=w164:errorcluster)  [unwired: 12 in]
                        "Galvo" <- TRUE
                      }
                      frame #1 {
                        n78 = flat-sequence {
                          tunnel: [w200] -> w193
                          tunnel: w192 -> [w198]
                          tunnel: [w197] -> w191
                          tunnel: w184 -> [w196]
                          tunnel: w183 -> [w195]
                          tunnel: w182 -> [w194]
                          tunnel: [w194] -> w181
                          tunnel: [w218] -> w189
                          tunnel: w193 -> [w216]
                          tunnel: w191 -> [w217]
                          tunnel: [w217] -> w190
                          tunnel: [FALSE ("Galvo")] -> w188
                          tunnel: w181 -> [w214]
                          tunnel: [w213] -> w180
                          frame #0 {
                            n79 = case shown="No Error" w196 {
                              tunnel: [w208 w210] -> w200
                              tunnel: [w207 w211] -> w197
                              tunnel: [w206 FALSE ("SaveStatus")] -> w199
                              tunnel: w198 -> [w205 w211]
                              tunnel: w196 -> [w202 w210]
                              tunnel: w195 -> [w201 _]
                              frame No Error {
                                n80 = local read "AcqSet"() -> (w204:T9)
                                n81 = Unbundle By Name(w204) -> ("KineticNum"=w203:i32)
                                n82 = local read "FilePath"() -> (w209:string)
                                n83 = Increment(x=w205) -> (x+1=w207:i32)
                                n84 = call "AndorSaveasSif_Ver2.vi"("Time"=w201, "error in"=w202, "No."=w205, "KinNumber"=w203, "FilePath"=w209) -> ("error out"=w208:errorcluster, "SaveStatus"=w206:bool)  [unwired: 5 in]
                                "CurrentFrame" <- w205
                              }
                              frame Error {
                              }
                            }
                            n85 = local write "SaveStatus"(w199) -> ()
                          }
                          frame #1 {
                            n86 = flat-sequence {
                              tunnel: [w226] -> w220
                              tunnel: [TRUE] -> w219
                              tunnel: w216 -> [w224]
                              tunnel: [w222] -> w213
                              tunnel: w214 -> [w221]
                              frame #0 {
                                n87 = call <vilib>:"DAQmx Start Task.vi"("task/channels in"=w221, "error in"=w224) -> ("task out"=w222:refnum<k21>, "error out"=w223:errorcluster)  [unwired: 12 in]
                                n88 = call <userlib>:"StartAcquisition.vi"("error in (no error)"=w223) -> ("error out"=w226:errorcluster)  [unwired: 1 in, 1 out]
                              }
                            }
                            n89 = local write "Andor"(w219) -> ()
                            n90 = while {
                              tunnel: w220 -> [w231]
                              tunnel: [w228] -> w218
                              stop <- w227 continue-if-true
                              n91 = call <userlib>:"GetStatus.vi"("error in (no error)"=w231) -> ("error out"=w228:errorcluster, "status"=w230:T20)  [unwired: 2 in, 1 out]
                              n92 = Equal?(x=Error_Code_Enum_typedef."DRV_ACQUIRING" ("y"), y=w230) -> (x = y?=w227:bool)
                              "Andor" <- w227
                            }
                          }
                        }
                        n93 = local write "Galvo"(w188) -> ()
                      }
                    }
                    "V" <- w142
                  }
                  "H" <- w126
                }
                n94 = local write "Galvo"(w113) -> ()
                n95 = call <vilib>:"DAQmx Stop Task.vi"("task/channels in"=w111, "error in"=w110) -> ("task out"=w108:refnum<k21>, "error out"=w109:errorcluster)  [unwired: 12 in]
              }
              event "Galvo Stop": Value Change {
                (unwired) T19."Disabled and Grayed Out" ("Disabled")
                w233 = T19."Enabled" ("Disabled")
                n96 = event-data() -> ()  [unwired: 1 in, 6 out]
                n97 = property on="Galvo Scan" class="Bool"("DisabledEnum"=w233) -> ()  [unwired: 2 in, 2 out]
                n98 = property on="Galvo Center" class="Bool"("DisabledEnum"=w233) -> ()  [unwired: 2 in, 2 out]
              }
            }
          }
        }
      }
      n99 = call <vilib>:"Simple Error Handler.vi"("error in (no error)"=w2) -> ()  [unwired: 4 in, 5 out]
    }
  }
  n100 = while {
    stop <- w236 stop-if-true
    n101 = local read "Initialization finished"() -> (w237:bool)
    n102 = case shown="True" w237 {
      tunnel: [FALSE ("ShutDown") w240] -> w236
      frame False {
      }
      frame True {
        n103 = while {
          shift-right: [w248] -> _
          shift-left: enum16{"Initialize", "Live", "Exit"}."Initialize" -> [w249]
          shift-right: [w246] -> _
          shift-left: errorcluster {"status"=FALSE, "code"=0, "source"=""} ("error in") -> [w247]
          tunnel: [w245] -> w240
          shift-right: [w243] -> _
          shift-left: TRUE -> [w244]
          stop <- w245 stop-if-true
          n104 = case shown="\"Live\"" w249 {
            tunnel: [enum16{"Initialize", "Live", "Exit"}."Live" w296 enum16{"Initialize", "Live", "Exit"}."Exit"] -> w248
            tunnel: w247 -> [w255 w295 w369]
            tunnel: [w252 w294 w368] -> w246
            tunnel: [FALSE ("ShutDown") FALSE ("ShutDown") w360] -> w245
            tunnel: w244 -> [w250 w291 w359]
            tunnel: [w250 w290 w359] -> w243
            frame "Initialize", Default {
              n105 = flat-sequence {
                tunnel: [w264] -> w256
                tunnel: w255 -> [w264]
                tunnel: w256 -> [w278]
                tunnel: [w277] -> w254
                tunnel: w254 -> [w286]
                tunnel: [w285] -> w253
                tunnel: w253 -> [w289]
                tunnel: [w289] -> w252
                frame #0 {
                  n106 = local write "ShutDown"(cluster{"CoolOff":bool, "ShutDown":bool} {"CoolOff"=FALSE, "ShutDown"=FALSE} ("ShutDown")) -> ()
                  n107 = local write "SetStatus"(FALSE ("SetStatus")) -> ()
                  n108 = local write "GetStatus"(T16 {"GetDetector"=FALSE, "GetHardVer"=FALSE, "GetNVS"=FALSE, "GetVS"=FALSE, "GetSotfVer"=FALSE, "GetNHS"=FALSE, "GetHS"=FALSE} ("GetStatus")) -> ()
                  n109 = local write "SaveStatus"(FALSE ("Save")) -> ()
                  n110 = local write "CoolerON"(T15 {"SetTemp"=FALSE, "CoolerOn"=FALSE, "Stablized"=FALSE} ("CoolerON")) -> ()
                  n111 = local write "DevInit"(FALSE ("DevInit")) -> ()
                }
                frame #1 {
                  n112 = local read "TargetTemp"() -> (w273:i32)
                  n113 = control-ref of="CurrentTemp"() -> (w275:refnum<vi>)
                  n114 = control-ref of="GetStatus"() -> (w276:refnum<vi>)
                  n115 = control-ref of="CoolerON"() -> (w274:refnum<vi>)
                  n116 = call "AndorInit.vi"("TargetTemp"=w273, "error in"=w278, "CoolerONRef"=w274, "GetStatusRef"=w276, "CurrentTempRef"=w275) -> ("GetStatus"=w265:T16, "CurrentTemp"=w272:i32, "CoolerON"=w271:T15, "DevInit"=w268:bool, "DevSize"=w267:cluster{"xpixels":i32, "ypixels":i32}, "HardWVersion"=w266:T12, "SoftWVersion"=w269:T13, "Speeds"=w270:T14, "error out"=w277:errorcluster)  [unwired: 6 in]
                  n117 = local write "CurrentTemp"(w272) -> ()
                  n118 = local write "SoftWVersion"(w269) -> ()
                  n119 = local write "Speeds"(w270) -> ()
                  n120 = local write "HardWVersion"(w266) -> ()
                  n121 = local write "DevSize"(w267) -> ()
                  n122 = local write "DevInit"(w268) -> ()
                  n123 = local write "GetStatus"(w265) -> ()
                  n124 = local write "CoolerON"(w271) -> ()
                }
                frame #2 {
                  n125 = local read "MultiTrack"() -> (w282:cluster{"StartRow":i32, "EndRow":i32})
                  n126 = local read "AcqSet"() -> (w284:T9)
                  n127 = local read "Mode"() -> (w283:T8)
                  n128 = call "AndorSet.vi"("error in"=w286, "MultiTrack"=w282, "AcqSet"=w284, "Mode"=w283) -> ("error out"=w285:errorcluster, "SetStatus"=w279:bool, "SetOut"=w280:T11, "Timing"=w281:T10)  [unwired: 4 in]
                  n129 = local write "SetOut"(w280) -> ()
                  n130 = local write "Timing"(w281) -> ()
                  n131 = local write "SetStatus"(w279) -> ()
                }
                frame #3 {
                  n132 = call "Display Message to User2"("Enable"=TRUE, "Message"="Andor now is ready!!!") -> ()  [unwired: 8 in, 2 out]
                }
              }
            }
            frame "Live" {
              n133 = event shown="[0] Timeout" {
                selector: _ -> [_ _ _ _ _ _]
                dyn-events: _ -> [_ _ _ _ _ _]
                timeout: 0 -> [_ _ _ _ _ _]
                tunnel: [enum16{"Initialize", "Live", "Exit"}."Live" enum16{"Initialize", "Live", "Exit"}."Live" enum16{"Initialize", "Live", "Exit"}."Live" enum16{"Initialize", "Live", "Exit"}."Live" enum16{"Initialize", "Live", "Exit"}."Live" enum16{"Initialize", "Live", "Exit"}."Exit"] -> w296
                tunnel: w295 -> [w299 w308 w315 w327 w332 w357]
                tunnel: [w298 w308 w315 w326 w330 w357] -> w294
                tunnel: w291 -> [w297 w306 w313 w319 w329 w356]
                tunnel: [w297 w305 w312 w319 w329 w356] -> w290
                event Timeout {
                  n134 = event-data() -> ()  [unwired: 1 in, 3 out]
                  n135 = Wait Until Next ms Multiple(millisecond multiple=u32 500) -> ()  [unwired: 1 out]
                  n136 = case shown="False" w297 {
                    tunnel: w299 -> [w302 w303]
                    tunnel: [w302 w303] -> w298
                    frame False {
                    }
                    frame True {
                      n137 = call <userlib>:"GetTemperature.vi"("error in (no error)"=w303) -> ("temperature"=w304:i32)  [unwired: 3 in, 3 out]
                      n138 = local write "CurrentTemp"(w304) -> ()
                    }
                  }
                }
                event "Galvo Scan": Value Change {
                  n139 = event-data() -> ()  [unwired: 1 in, 6 out]
                  n140 = case shown="True" w306 {
                    tunnel: w306 -> [w309 w311]
                    tunnel: [w309 w310] -> w305
                    frame False {
                    }
                    frame True {
                      n141 = Not(x=w311) -> (.not. x?=w310:bool)
                    }
                  }
                }
                event "Galvo Stop": Value Change {
                  n142 = event-data() -> ()  [unwired: 1 in, 6 out]
                  n143 = case shown="False" w313 {
                    tunnel: w313 -> [w317 w318]
                    tunnel: [w316 w318] -> w312
                    frame False {
                      n144 = Not(x=w317) -> (.not. x?=w316:bool)
                    }
                    frame True {
                    }
                  }
                }
                event "Set": Value Change {
                  n145 = event-data() -> ()  [unwired: 1 in, 6 out]
                  n146 = local read "AcqSet"() -> (w324:T9)
                  n147 = local read "MultiTrack"() -> (w323:cluster{"StartRow":i32, "EndRow":i32})
                  n148 = local read "Mode"() -> (w325:T8)
                  n149 = call "AndorSet.vi"("error in"=w327, "MultiTrack"=w323, "AcqSet"=w324, "Mode"=w325) -> ("error out"=w326:errorcluster, "SetStatus"=w321:bool, "SetOut"=w320:T11, "Timing"=w322:T10)  [unwired: 4 in]
                  n150 = local write "Timing"(w322) -> ()
                  n151 = local write "SetStatus"(w321) -> ()
                  n152 = local write "SetOut"(w320) -> ()
                }
                event "AndorSnap": Value Change {
                  n153 = event-data() -> ()  [unwired: 1 in, 6 out]
                  n154 = flat-sequence {
                    tunnel: [w335] -> w333
                    tunnel: w332 -> [w338]
                    tunnel: w333 -> [w350]
                    tunnel: [TRUE ("SaveStatus")] -> w331
                    tunnel: [w347] -> w330
                    frame #0 {
                      n155 = case shown="No Error" w338 {
                        tunnel: w338 -> [w341 w346]
                        tunnel: [w340 FALSE ("SaveStatus")] -> w337
                        tunnel: [w339 w346] -> w335
                        frame No Error {
                          n156 = local read "AcqSet"() -> (w343:T9)
                          n157 = Unbundle By Name(w343) -> ("KineticNum"=w342:i32)
                          n158 = call "AndorSaveasSif.vi"("error in"=w341, "KinNumber"=w342, "FilePath"="FilePath") -> ("error out"=w339:errorcluster, "SaveStatus"=w340:bool)  [unwired: 7 in]
                        }
                        frame Error {
                        }
                      }
                      n159 = Not(x=w337) -> (.not. x?=→"SaveStatus":bool)
                    }
                    frame #1 {
                      n160 = call <userlib>:"StartAcquisition.vi"("error in (no error)"=w350) -> ("error out"=w349:errorcluster)  [unwired: 1 in, 1 out]
                      n161 = while {
                        tunnel: w349 -> [w355]
                        tunnel: [w352] -> w347
                        stop <- w351 continue-if-true
                        n162 = call <userlib>:"GetStatus.vi"("error in (no error)"=w355) -> ("error out"=w352:errorcluster, "status"=w354:T20)  [unwired: 2 in, 1 out]
                        n163 = Equal?(x=w354, y=Error_Code_Enum_typedef."DRV_ACQUIRING") -> (x = y?=w351:bool)
                      }
                    }
                  }
                  n164 = local write "SaveStatus"(w331) -> ()
                }
                event "Exit": Value Change {
                  n165 = event-data() -> ()  [unwired: 1 in, 6 out]
                }
              }
            }
            frame "Exit" {
              n166 = local read "CoolerON"() -> (w367:T15)
              n167 = Unbundle By Name(w367) -> ("SetTemp"=w366:bool, "CoolerOn"=w365:bool)
              n168 = control-ref of="CurrentTemp"() -> (w364:refnum<vi>)
              n169 = control-ref of="ShutDown"() -> (w362:refnum<vi>)
              n170 = call "AndorShutdown.vi"("ShutDownRef"=w362, "CurrentTempRef"=w364, "error in"=w369, "CoolerON"=w365, "SetTemp"=w366) -> ("error out"=w368:errorcluster, "ShutDown"=w361:cluster{"CoolOff":bool, "ShutDown":bool}, "CurrentTemp"=w363:i32)  [unwired: 4 in]
              "ShutDown" <- w361
              n171 = local write "CurrentTemp"(w363) -> ()
              n172 = Unbundle By Name(w361) -> ("ShutDown"=w360:bool)  [unwired: 1 out]
            }
          }
        }
      }
    }
  }
